vi "MySubVI.vi"(1 "Wave Form":i16(ring) items=["Square", "Sawtooth", "Triangulaire", "Sine wave", "DC"], 2 "Freq. Unit":u16(ring) items=["mHz", "Hz", "kHz"], 3 "Duty Cycle (%)":dbl(knob) scale=0.0..100.0, 4 "Phase":dbl(slide) scale=-180.0..180.0, 5 "Offset":dbl(slide) scale=-5.0..5.0, 6 "Ampl.":dbl(knob) scale=0.0..5.0, 7 "Freq.":dbl(knob) scale=1.0..450.0) -> (0 "Waveform Graph":waveform(dbl)(graph))   [LabVIEW 2011]
uses:
  <vilib>/measure/NI_MABase.lvlib
  <vilib>/measure/NI_MAPro.lvlib
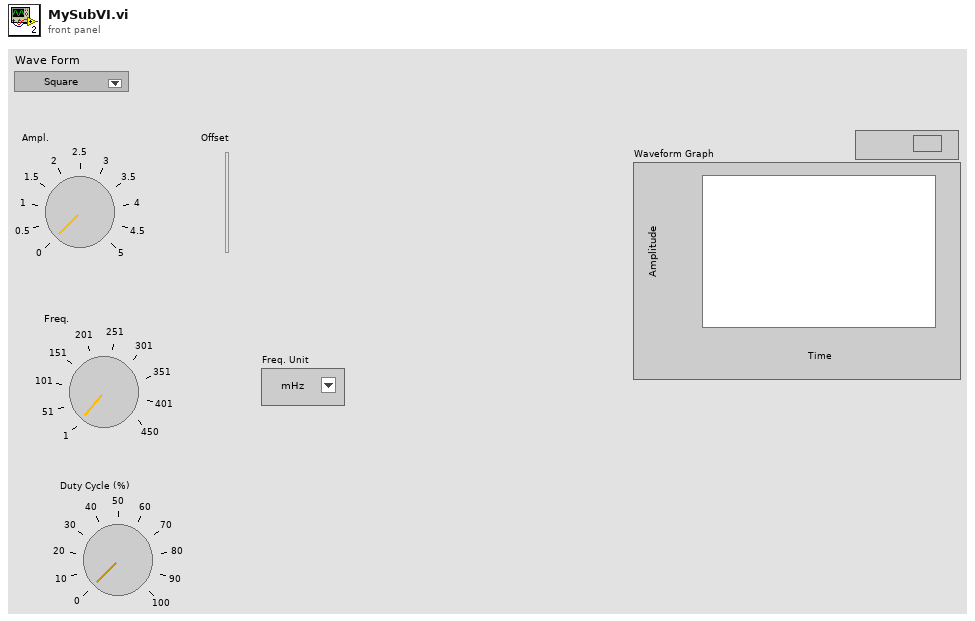
[diagram p1: front panel]
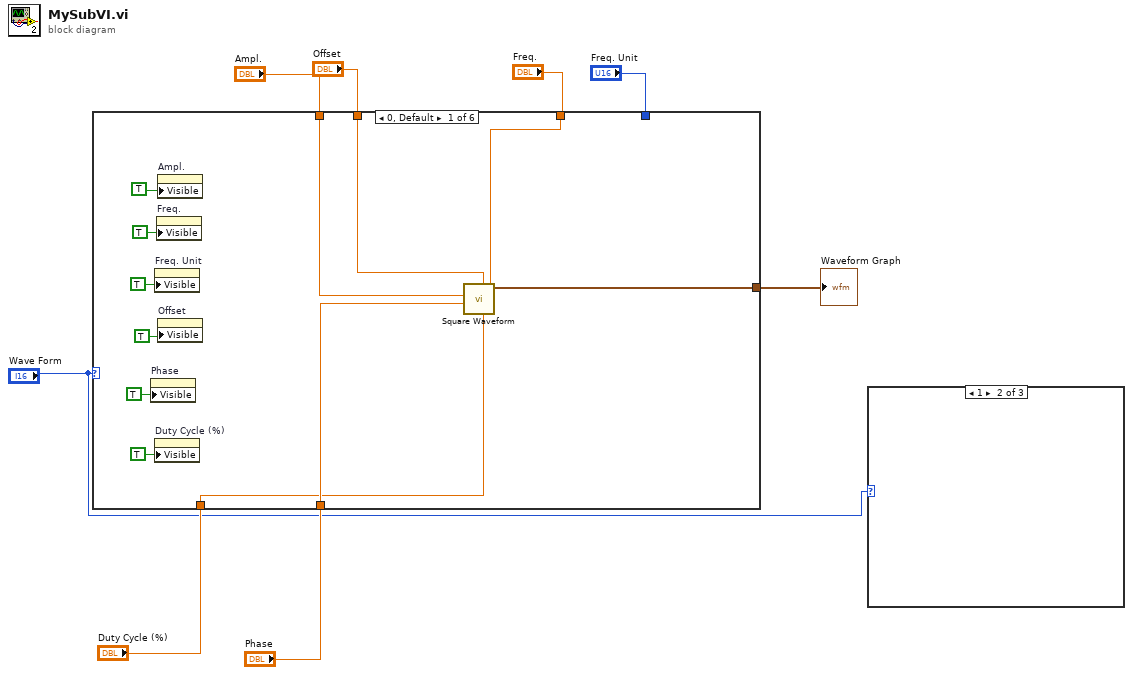
[diagram p0: block diagram]
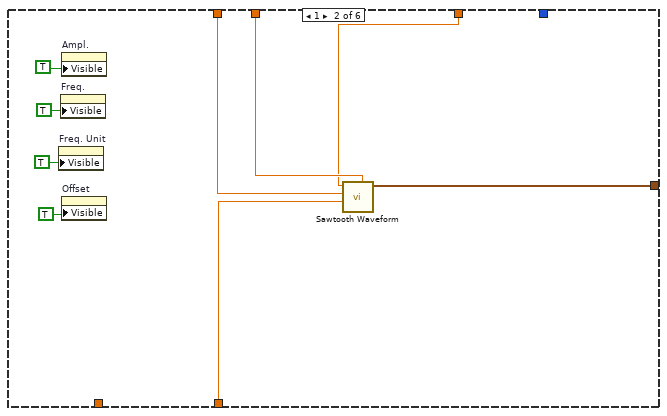
[diagram p4: hidden frame]
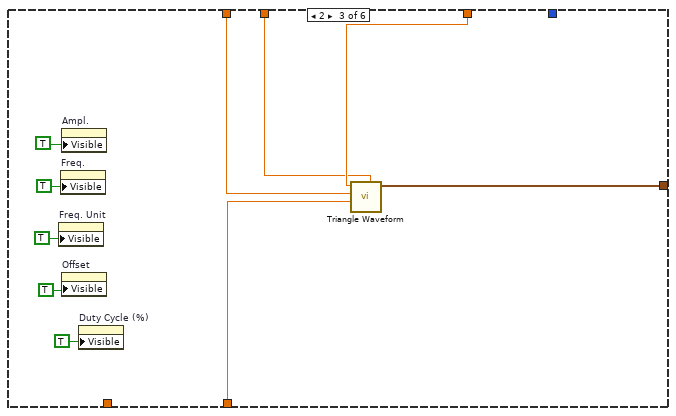
[diagram p5: hidden frame]
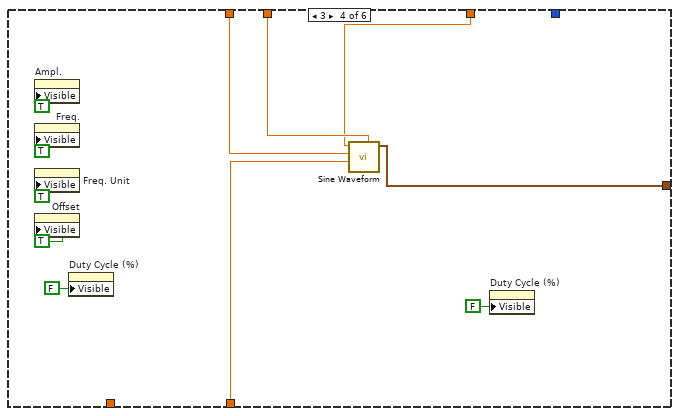
[diagram p6: hidden frame]
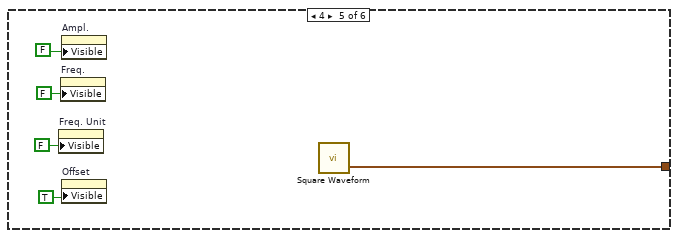
[diagram p7: hidden frame]
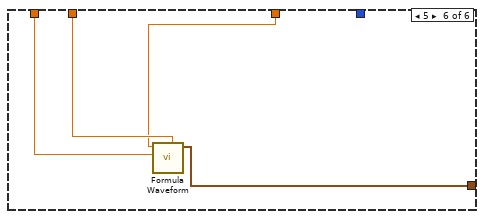
[diagram p8: hidden frame]
diagram:
  n1 = case shown="0, Default" "Wave Form" {
    tunnel: "Ampl." -> [w14 w23 w34 w44 _ w58]
    tunnel: "Freq. Unit" -> [_ _ _ _ _ _]
    tunnel: "Freq." -> [w15 w24 w35 w43 _ w57]
    tunnel: "Offset" -> [w16 w25 w33 w46 _ w59]
    tunnel: "Phase" -> [w11 w22 w32 w45 _ _]
    tunnel: "Duty Cycle (%)" -> [w10 _ _ _ _ _]
    tunnel: [w9 w21 w31 w42 w51 w56] -> w2
    frame 0, Default {
      n2 = property on="Phase" class="Slide (strict)"("Visible"=TRUE) -> ()  [unwired: 2 in, 2 out]
      n3 = property on="Freq. Unit" class="Ring (strict)"("Visible"=TRUE) -> ()  [unwired: 2 in, 2 out]
      n4 = property on="Duty Cycle (%)" class="Knob (strict)"("Visible"=TRUE) -> ()  [unwired: 2 in, 2 out]
      n5 = property on="Freq." class="Knob (strict)"("Visible"=TRUE) -> ()  [unwired: 2 in, 2 out]
      n6 = property on="Ampl." class="Knob (strict)"("Visible"=TRUE) -> ()  [unwired: 2 in, 2 out]
      n7 = property on="Offset" class="Slide (strict)"("Visible"=TRUE) -> ()  [unwired: 2 in, 2 out]
      n8 = call <vilib>:"Square Waveform.vi"("duty cycle (%)"=w10, "offset"=w16, "phase"=w11, "amplitude"=w14, "frequency"=w15) -> ("signal out"=w9:waveform(dbl))  [unwired: 5 in, 1 out]
    }
    frame 1 {
      n9 = property on="Freq. Unit" class="Ring (strict)"("Visible"=TRUE) -> ()  [unwired: 2 in, 2 out]
      n10 = property on="Freq." class="Knob (strict)"("Visible"=TRUE) -> ()  [unwired: 2 in, 2 out]
      n11 = property on="Ampl." class="Knob (strict)"("Visible"=TRUE) -> ()  [unwired: 2 in, 2 out]
      n12 = property on="Offset" class="Slide (strict)"("Visible"=TRUE) -> ()  [unwired: 2 in, 2 out]
      n13 = call <vilib>:"Sawtooth Waveform.vi"("offset"=w25, "phase"=w22, "amplitude"=w23, "frequency"=w24) -> ("signal out"=w21:waveform(dbl))  [unwired: 6 in, 1 out]
    }
    frame 2 {
      n14 = property on="Freq. Unit" class="Ring (strict)"("Visible"=TRUE) -> ()  [unwired: 2 in, 2 out]
      n15 = property on="Freq." class="Knob (strict)"("Visible"=TRUE) -> ()  [unwired: 2 in, 2 out]
      n16 = property on="Ampl." class="Knob (strict)"("Visible"=TRUE) -> ()  [unwired: 2 in, 2 out]
      n17 = property on="Offset" class="Slide (strict)"("Visible"=TRUE) -> ()  [unwired: 2 in, 2 out]
      n18 = property on="Duty Cycle (%)" class="Knob (strict)"("Visible"=TRUE) -> ()  [unwired: 2 in, 2 out]
      n19 = call <vilib>:"Triangle Waveform.vi"("offset"=w33, "phase"=w32, "amplitude"=w34, "frequency"=w35) -> ("signal out"=w31:waveform(dbl))  [unwired: 6 in, 1 out]
    }
    frame 3 {
      n20 = property on="Ampl." class="Knob (strict)"("Visible"=TRUE) -> ()  [unwired: 2 in, 2 out]
      n21 = property on="Freq." class="Knob (strict)"("Visible"=TRUE) -> ()  [unwired: 2 in, 2 out]
      n22 = property on="Freq. Unit" class="Ring (strict)"("Visible"=TRUE) -> ()  [unwired: 2 in, 2 out]
      n23 = property on="Offset" class="Slide (strict)"("Visible"=TRUE) -> ()  [unwired: 2 in, 2 out]
      n24 = property on="Duty Cycle (%)" class="Knob (strict)"("Visible"=FALSE) -> ()  [unwired: 2 in, 2 out]
      n25 = call <vilib>:"Sine Waveform.vi"("offset"=w46, "phase"=w45, "amplitude"=w44, "frequency"=w43) -> ("signal out"=w42:waveform(dbl))  [unwired: 6 in, 1 out]
      n26 = property on="Duty Cycle (%)" class="Knob (strict)"("Visible"=FALSE) -> ()  [unwired: 2 in, 2 out]
    }
    frame 4 {
      n27 = property on="Freq. Unit" class="Ring (strict)"("Visible"=FALSE) -> ()  [unwired: 2 in, 2 out]
      n28 = property on="Freq." class="Knob (strict)"("Visible"=FALSE) -> ()  [unwired: 2 in, 2 out]
      n29 = property on="Ampl." class="Knob (strict)"("Visible"=FALSE) -> ()  [unwired: 2 in, 2 out]
      n30 = property on="Offset" class="Slide (strict)"("Visible"=TRUE) -> ()  [unwired: 2 in, 2 out]
      n31 = call <vilib>:"Square Waveform.vi"() -> ("signal out"=w51:waveform(dbl))  [unwired: 10 in, 1 out]
    }
    frame 5 {
      n32 = call <vilib>:"Formula Waveform.vi"("offset"=w59, "amplitude"=w58, "frequency"=w57) -> ("signal out"=w56:waveform(dbl))  [unwired: 7 in, 1 out]
    }
  }
  "Waveform Graph" <- w2
  n33 = case shown="1" "Wave Form" {
    frame 0, Default {
    }
    frame 1 {
    }
    frame 2 {
    }
  }
